vi "Create User Events.vi"(8 "Error In":errorcluster) -> (0 "Error Out":errorcluster, 1 "PS4 Event Refs":refnum<event-registration>, 2 "Events":T1)   [LabVIEW 2020, in "LMH-PS4.lvlib"]
uses:
  LMH-PS4.lvlib
  Type Defs/PS4 Button Events.ctl
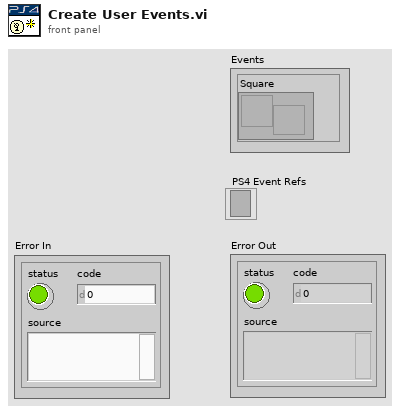
[diagram p1: front panel]
types:
  T1 = typedef "LMH-PS4.lvlib/PS4 Button Events.ctl" = cluster{"Square":refnum<user-event>, "X":refnum<user-event>, "Circle":refnum<user-event>, "Triangle":refnum<user-event>, "L1":refnum<user-event>, "R1":refnum<user-event>, "L2":refnum<user-event>, "R2":refnum<user-event>, "Share":refnum<user-event>, "Options":refnum<user-event>, "Left Thumbstick":refnum<user-event>, "Right Thumbstick":refnum<user-event>, "Playstation Button":refnum<user-event>, "Pad":refnum<user-event>}
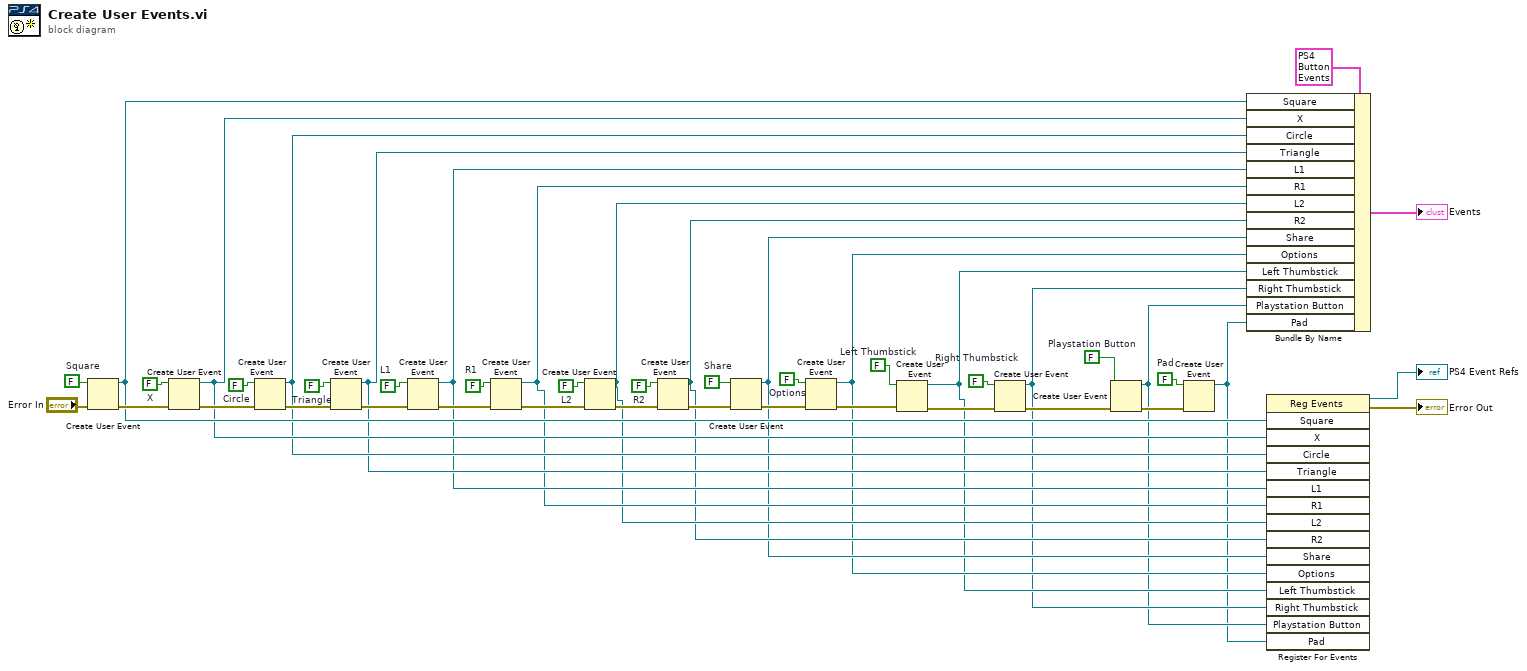
[diagram p0: block diagram]
diagram:
  w22 = FALSE  # Pad
  w23 = FALSE  # Playstation Button
  w24 = FALSE  # Right Thumbstick
  w25 = FALSE  # Left Thumbstick
  w34 = FALSE  # Options
  w35 = FALSE  # Share
  w38 = FALSE  # R2
  w39 = FALSE  # L2
  w40 = FALSE  # R1
  w41 = FALSE  # L1
  w42 = FALSE  # Triangle
  w43 = FALSE  # Circle
  w45 = FALSE  # X
  w44 = FALSE  # Square
  n1 = Create User Event(user event datatype=w44, error in="Error In") -> (user event=w17:refnum<user-event>, error out=w37:errorcluster)
  n2 = Create User Event(user event datatype=w45, error in=w37) -> (user event=w16:refnum<user-event>, error out=w36:errorcluster)
  n3 = Create User Event(user event datatype=w43, error in=w36) -> (user event=w15:refnum<user-event>, error out=w33:errorcluster)
  n4 = Create User Event(user event datatype=w42, error in=w33) -> (user event=w14:refnum<user-event>, error out=w32:errorcluster)
  n5 = Create User Event(user event datatype=w41, error in=w32) -> (user event=w13:refnum<user-event>, error out=w31:errorcluster)
  n6 = Create User Event(user event datatype=w40, error in=w31) -> (user event=w12:refnum<user-event>, error out=w30:errorcluster)
  n7 = Create User Event(user event datatype=w39, error in=w30) -> (user event=w11:refnum<user-event>, error out=w29:errorcluster)
  n8 = Create User Event(user event datatype=w38, error in=w29) -> (user event=w10:refnum<user-event>, error out=w28:errorcluster)
  n9 = Create User Event(user event datatype=w35, error in=w28) -> (user event=w9:refnum<user-event>, error out=w27:errorcluster)
  n10 = Create User Event(user event datatype=w34, error in=w27) -> (user event=w8:refnum<user-event>, error out=w21:errorcluster)
  n11 = Create User Event(user event datatype=w25, error in=w21) -> (user event=w7:refnum<user-event>, error out=w20:errorcluster)
  n12 = Create User Event(user event datatype=w24, error in=w20) -> (user event=w6:refnum<user-event>, error out=w19:errorcluster)
  n13 = Create User Event(user event datatype=w23, error in=w19) -> (user event=w5:refnum<user-event>, error out=w18:errorcluster)
  n14 = Create User Event(user event datatype=w22, error in=w18) -> (user event=w4:refnum<user-event>)  [unwired: 1 out]
  n15 = Bundle By Name(cluster=T1 {"Square"=refnum, "X"=refnum, "Circle"=refnum, "Triangle"=refnum, "L1"=refnum, "R1"=refnum, "L2"=refnum, "R2"=refnum, "Share"=refnum, "Options"=refnum, "Left Thumbstick"=refnum, "Right Thumbstick"=refnum, "Playstation Button"=refnum, "Pad"=refnum} ("output cluster"), "Square"=w17, "X"=w16, "Circle"=w15, "Triangle"=w14, "L1"=w13, "R1"=w12, "L2"=w11, "R2"=w10, "Share"=w9, "Options"=w8, "Left Thumbstick"=w7, "Right Thumbstick"=w6, "Playstation Button"=w5, "Pad"=w4) -> (→"Events":T1)
  n16 = register-events(w17, w16, w15, w14, w13, w12, w11, w10, w9, w8, w7, w6, w5, w4) -> (reference out=→"PS4 Event Refs":refnum<event-registration>, error out=→"Error Out":errorcluster)  [unwired: 2 in]
